vi "dfd_Merge NStage FLP and FXP Analysis Outputs.vi"(7 "output option":u16(ring) items=["Auto", "Floating-point Only", "Fixed-point Only"], 8 "error in FXP":errorcluster, 9 "freq response":cluster{"f0":dbl, "df":dbl, "values":dbl[]}[](graph), 10 "error in FLP":errorcluster, 11 "freq response":cluster{"f0":dbl, "df":dbl, "values":dbl[]}[](graph)) -> (0 "error out":errorcluster, 3 "freq response":cluster{"f0":dbl, "df":dbl, "values":dbl[]}[](graph))   [LabVIEW 2017, in "NI_DigFilterLicensed.lvlib"]
uses:
  <vilib>/addons/Digital Filter Design/NI_DigFilterLicensed.lvlib
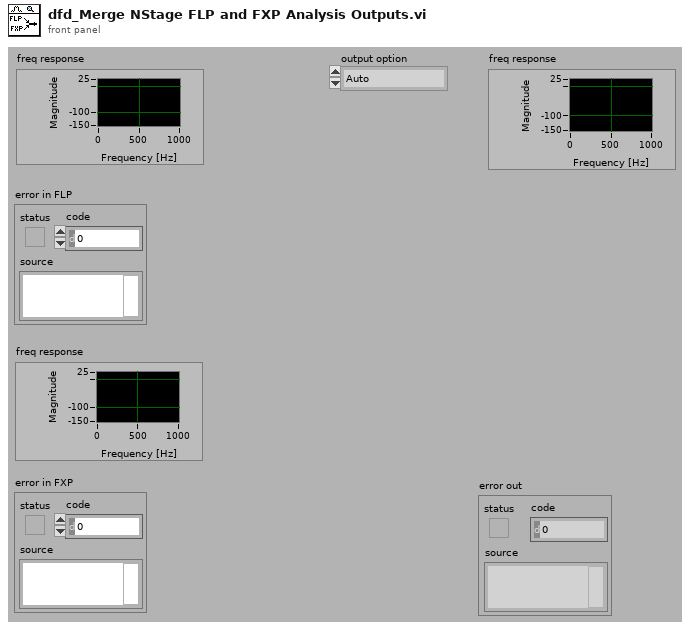
[diagram p1: front panel]
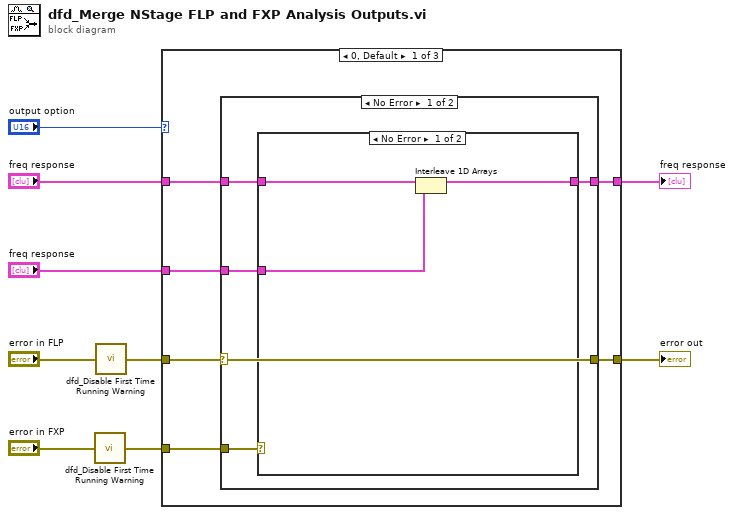
[diagram p0: block diagram]
diagram:
  n1 = call <vilib>:"dfd_Disable First Time Running Warning.vi"("error in"="error in FXP") -> ("error out"=w4:errorcluster)  [unwired: 1 in]
  n2 = call <vilib>:"dfd_Disable First Time Running Warning.vi"("error in"="error in FLP") -> ("error out"=w6:errorcluster)  [unwired: 1 in]
  n3 = case shown="0, Default" "output option" {
    tunnel: "freq response" -> [w13 w26 _]
    tunnel: "freq response" -> [w11 _ w28]
    tunnel: w6 -> [w15 w27 _]
    tunnel: w4 -> [w14 _ w29]
    tunnel: [w12 w26 w28] -> w3
    tunnel: [w10 w27 w29] -> w7
    frame 0, Default {
      n4 = case shown="No Error" w15 {
        selector: w15 -> [w16 w25]
        tunnel: w14 -> [w20 _]
        tunnel: w13 -> [w19 _]
        tunnel: [w18 _] -> w12
        tunnel: w11 -> [w17 _]
        tunnel: [w16 w25] -> w10
        frame No Error {
          n5 = case shown="No Error" w20 {
            tunnel: w19 -> [w23 w24]
            tunnel: [w21 w24] -> w18
            tunnel: w17 -> [w22 _]
            frame No Error {
              n6 = Interleave 1D Arrays(w23, w22) -> (w21:cluster{"f0":dbl, "df":dbl, "values":dbl[]}[])
            }
            frame Error {
            }
          }
        }
        frame Error {
        }
      }
    }
    frame 1 {
    }
    frame 2 {
    }
  }
  "error out" <- w7
  "freq response" <- w3
